vi "Create Child for Two Point Crossover.vi"(8 "Cut Point Index 2":i32, 9 "Cut Point Index 1":i32, 10 "SCH 2":u16[](array[numeric]), 11 "SCH 1":u16[](array[numeric])) -> (3 "Child Out":u16[](array[numeric]))   [LabVIEW 2013, in "GA.lvclass"]
uses:
  GA.lvclass
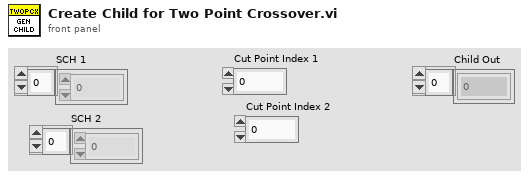
[diagram p1: front panel]
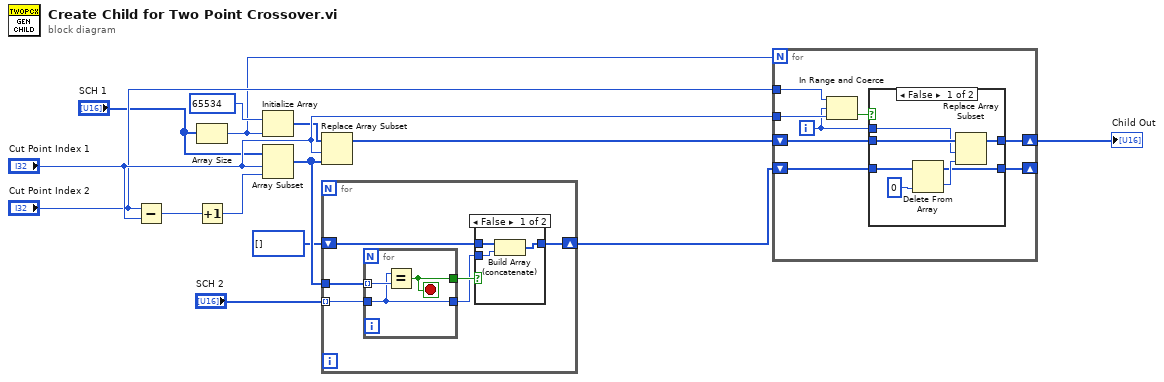
[diagram p0: block diagram]
diagram:
  n1 = Subtract(x="Cut Point Index 2", y="Cut Point Index 1") -> (x-y=w9:i32)
  n2 = Array Size(array="SCH 1") -> (size(s)=w1:i32)
  n3 = Increment(x=w9) -> (x+1=w8:i32)
  n4 = Initialize Array(u16 65534, w1) -> (w6:u16[])
  n5 = Array Subset(array="SCH 1", index="Cut Point Index 1", length=w8) -> (w5:u16[])
  n6 = Replace Array Subset(array=w6, new element=w5, index="Cut Point Index 1") -> (w3:u16[])
  n7 = for {
    tunnel: w5 -> [w19]
    tunnel: "SCH 2" -> [w20] mode=indexing
    shift-right: [w15] -> w2
    shift-left: u16[] [] -> [w16]
    n8 = for {
      tunnel: w20 -> [w25]
      tunnel: w19 -> [w27] mode=indexing
      tunnel: [w26] -> w18
      tunnel: [w25] -> w17
      stop <- w26 stop-if-true
      n9 = Equal?(x=w25, y=w27) -> (x = y?=w26:bool)
    }
    n10 = case shown="False" w18 {
      tunnel: w17 -> [w22 _]
      tunnel: w16 -> [w23 w24]
      tunnel: [w21 w24] -> w15
      frame False {
        n11 = Build Array (concatenate)(w23, w22) -> (w21:u16[])
      }
      frame True {
      }
    }
  }
  n12 = for {
    N: w1 -> [_]
    tunnel: "Cut Point Index 2" -> [w35]
    tunnel: "Cut Point Index 1" -> [w34]
    shift-right: [w29] -> w14
    shift-left: w3 -> [w32]
    shift-right: [w28] -> _
    shift-left: w2 -> [w30]
    i -> [w31]
    n13 = In Range and Coerce(upper limit=w35, x=w31, lower limit=w34) -> (In Range?=w33:bool)  [unwired: 1 out]
    n14 = case shown="False" w33 {
      tunnel: w32 -> [w42 w44]
      tunnel: w31 -> [w41 _]
      tunnel: w30 -> [w40 w43]
      tunnel: [w37 w44] -> w29
      tunnel: [w36 w43] -> w28
      frame False {
        n15 = Delete From Array(array=w40, index=0) -> (deleted portion=w38:u16, array with subset deleted=w36:u16[])  [unwired: 1 in]
        n16 = Replace Array Subset(array=w42, new element=w38, index=w41) -> (w37:u16[])
      }
      frame True {
      }
    }
  }
  "Child Out" <- w14
